vi "PH_Beamline.color Beamline.vi"(0 "i ref in":refnum<vi>, 5 "error in (no error)":errorcluster) -> (14 "i ref out":refnum<vi>, 19 "error out":errorcluster)   [LabVIEW 2014, in "PH_Beamline.lvlib"]
doc: "This VI sets the color of several beamline elements."
uses:
  PH_Beamline.lvlib
  PH_BL-Master/PH_BL-Master.lvlib
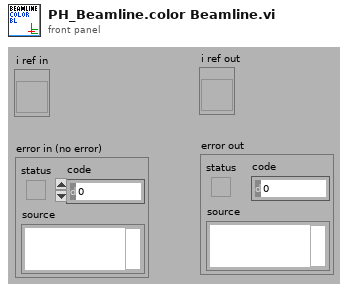
[diagram p1: front panel]
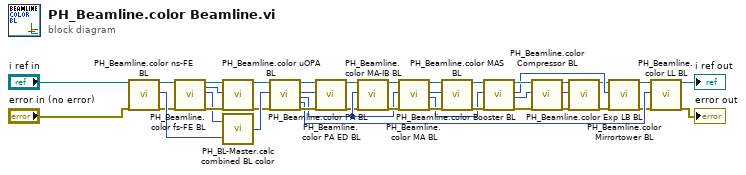
[diagram p0: block diagram]
diagram:
  n1 = call "PH_Beamline.color ns-FE BL.vi"("i ref in"="i ref in", "error in (no error)"="error in (no error)") -> ("i ref out"=w6:refnum<vi>, "Color State Exit ns-FE"=w32:i32, "error out"=w5:errorcluster)  [unwired: 15 in]
  n2 = call "PH_Beamline.color fs-FE BL.vi"("i ref in"=w6, "error in (no error)"=w5) -> ("i ref out"=w3:refnum<vi>, "Color State fs FE before Switch"=w1:i32, "Color State Exit fs-FE"=w31:i32, "error out"=w38:errorcluster)  [unwired: 14 in]
  n3 = call "PH_Beamline.color uOPA BL.vi"("i ref in"=w3, "Color State fs FE before Switch"=w1, "error in (no error)"=w38) -> ("i ref out"=w2:refnum<vi>, "error out"=w4:errorcluster)  [unwired: 15 in]
  n4 = call "PH_BL-Master.calc combined BL color.vi"("Color State BL 2"=w32, "Color State BL 1"=w31) -> ("Color State combined BL"=w13:i32)
  n5 = call "PH_Beamline.color PA BL.vi"("i ref in"=w2, "Color State PA Input"=w13, "error in (no error)"=w4) -> ("i ref out"=w35:refnum<vi>, "Color State PA Exit to ED"=w33:i32, "Color State PA Exit to MA"=w15:i32, "Color State PA Exit to Lab"=w14:i32, "error out"=w34:errorcluster)  [unwired: 12 in]
  n6 = call "PH_Beamline.color PA ED BL.vi"("i ref in"=w35, "Color State PA Exit to ED"=w33, "error in (no error)"=w34) -> ("i ref out"=w12:refnum<vi>, "error out"=w11:errorcluster)  [unwired: 15 in]
  n7 = call "PH_Beamline.color MA-IB BL.vi"("i ref in"=w12, "Color State MA Input"=w15, "error in (no error)"=w11) -> ("i ref out"=w40:refnum<vi>, "error out"=w39:errorcluster)  [unwired: 15 in]
  n8 = call "PH_Beamline.color MA BL.vi"("i ref in"=w40, "Color State MA Input"=w15, "error in (no error)"=w39) -> ("i ref out"=w29:refnum<vi>, "Color State MA Exit to MAS"=w28:i32, "Color State MA Exit to Booster"=w21:i32, "error out"=w30:errorcluster)  [unwired: 13 in]
  n9 = call "PH_Beamline.color MAS BL.vi"("i ref in"=w29, "Color State MAS Input"=w28, "error in (no error)"=w30) -> ("i ref out"=w25:refnum<vi>, "error out"=w23:errorcluster)  [unwired: 15 in]
  n10 = call "PH_Beamline.color Booster BL.vi"("i ref in"=w25, "Color State Booster Input"=w21, "error in (no error)"=w23) -> ("i ref out"=w24:refnum<vi>, "Color State Booster Exit to MT"=w19:i32, "Color State Booster Exit to Compressor"=w20:i32, "error out"=w22:errorcluster)  [unwired: 13 in]
  n11 = call "PH_Beamline.color Compressor BL.vi"("i ref in"=w24, "Color State Compressor Input"=w20, "error in (no error)"=w22) -> ("i ref out"=w27:refnum<vi>, "Color State Compressor Exit"=w16:i32, "error out"=w26:errorcluster)  [unwired: 14 in]
  n12 = call "PH_Beamline.color Exp LB BL.vi"("i ref in"=w27, "Color State Exp LB Input"=w16, "error in (no error)"=w26) -> ("i ref out"=w18:refnum<vi>, "error out"=w17:errorcluster)  [unwired: 15 in]
  n13 = call "PH_Beamline.color Mirrortower BL.vi"("i ref in"=w18, "Color State MT Input"=w19, "error in (no error)"=w17) -> ("i ref out"=w10:refnum<vi>, "error out"=w9:errorcluster)  [unwired: 14 in, 1 out]
  n14 = call "PH_Beamline.color LL BL.vi"("i ref in"=w10, "Color State Exp LB Input"=w14, "error in (no error)"=w9) -> ("i ref out"=→"i ref out":refnum<vi>, "error out"=→"error out":errorcluster)  [unwired: 15 in]
